vi "motor test 002.vi"() -> ()   [LabVIEW 2019]
uses:
  <vilib>/Platform/TimedLoop/XDataNode/timing_clust.ctl
  <vilib>/Platform/TimedLoop/XDataNode/nitl_modes.ctl
  <vilib>/Platform/TimedLoop/XDataNode/wakeup.ctl
  low level/motor/motor enum.ctl
  <vilib>/platform/TimedLoop/XDataNode/XDataNode.xnode
  low level/motor/motor.lvlib
  <vilib>/Platform/TimedLoop/XDataNode/XDNodeRunTimeDep.lvlib
panel:
  out "E":dbl
  out "Waveform Chart 2":dbl(graph)
  in  "PID gains":T1={"proportional gain (Kc)"=1800.0, "integral time (Ti, min)"=0.0, "derivative time (Td, min)"=0.012}
  out "Waveform Chart":dbl(graph)
  in  "speed RPM":dbl
  in  "reset":bool
  in  "Stop":bool
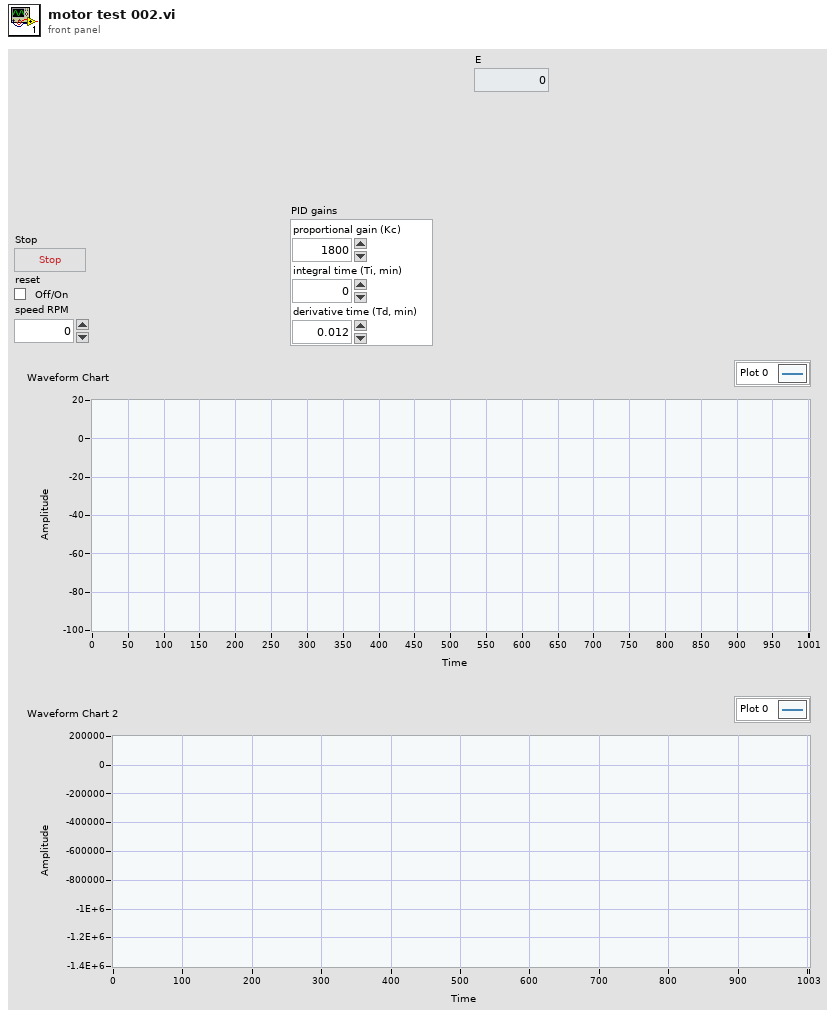
[diagram p1: front panel]
types:
  T1 = cluster{"proportional gain (Kc)":dbl, "integral time (Ti, min)":dbl, "derivative time (Td, min)":dbl}
  T2 = typedef "XDNodeRunTimeDep.lvlib/timing_clust.ctl" = cluster{"Expected End [f-1]":u64, "Actual End [f-1]":u64, "Finished Late? [f-1]":bool, "Expected End [i-1]":u64, "Actual End [i-1]":u64, "Finished Late? [i-1]":bool, "Expected Start [i]":u64, "Actual Start [i]":u64, "Expected Start [f]":u64, "Actual Start [f]":u64, "Source Name":string, "Structure Name":string, "Period":i64, "Deadline":i64, "Offset":i64, "Start":i64, "Priority":i32, "Timeout":i32, "Mode":T3, "Wakeup Reason":T4, "Error":errorcluster, "Source Type":string, "Secondary Source Type":string, "Global End Time":u64, "Global Start Time":u64, "Frame Duration":u64, "Iteration Duration":u64, "Assigned CPU":i32, "I/O Scan Engine Mode":u32}
  T3 = typedef "XDNodeRunTimeDep.lvlib/nitl_modes.ctl" = enum32{"No Change", "Process missed periods, maintain original phase", "Discard missed periods, maintain original phase", "Process missed periods, ignore original phase", "Discard missed periods, ignore original phase"}
  T4 = typedef "XDNodeRunTimeDep.lvlib/wakeup.ctl" = enum32{"Normal", "Aborted", "Asynchronous wakeup", "Timing source error", "Timed loop error", "Timeout"}
  T5 = typedef "my FPGA lib.lvlib/motor.lvlib/motor enum.ctl" = enum16{"M1", "M2", "M3", "M4"}
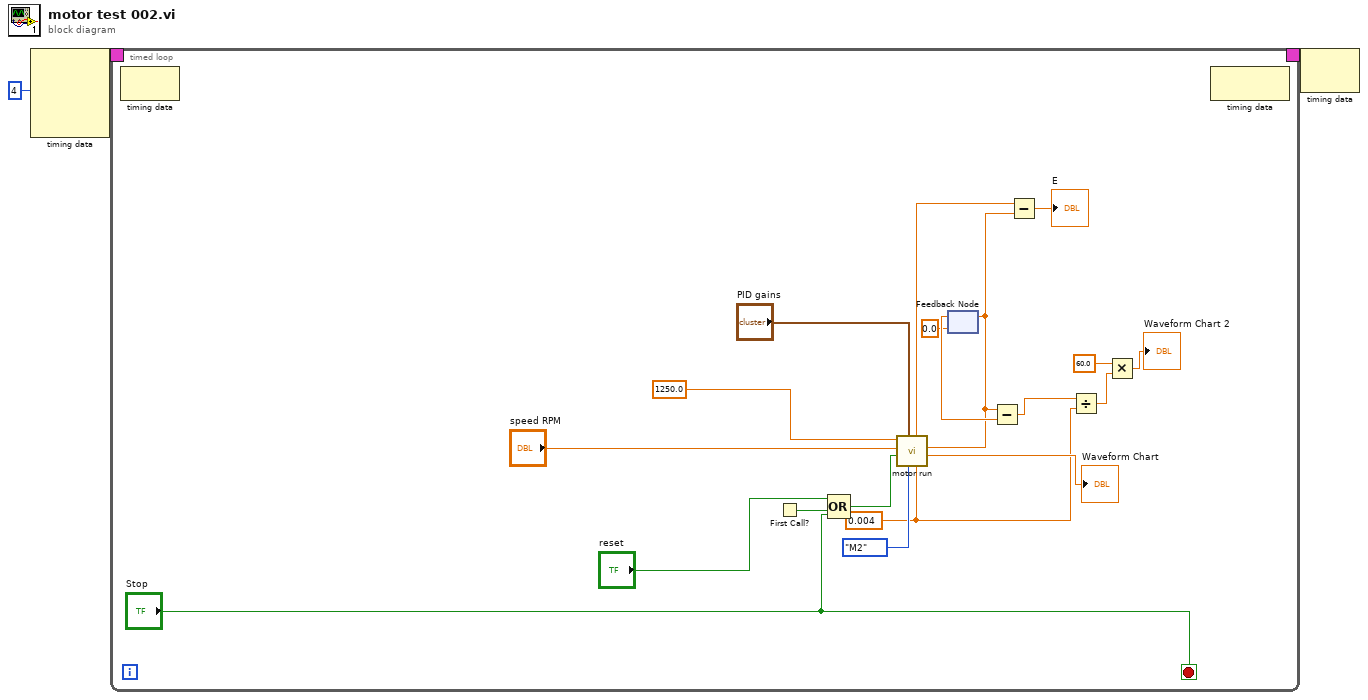
[diagram p0: block diagram]
diagram:
  n1 = node-c288(i64 4 ("Period")) -> (w3:T2)  [unwired: 3 in]
  n2 = timed-loop {
    timing: w3 -> [_]
    timing-out: [_] -> w2
    stop <- "Stop" stop-if-true
    w13 = 0.004 ("dt(s)")
    n3 = node-c288() -> ()  [unwired: 1 in, 1 out]
    n4 = First Call?() -> (First Call?: T/F=w21:bool)
    n5 = Compound Arithmetic op=OR("reset", w21, "Stop") -> (w19:bool)
    n6 = call "motor run.vi"("dt(s)"=w13, "motor select"=motor_enum."M2", "PID gains"="PID gains", "Reset"=w19, "speed RPM"="speed RPM", "PWM frequence"=1250.0) -> ("output"=→"Waveform Chart":dbl, "encoder"=w5:dbl, "setpoint"=w6:dbl)  [unwired: 2 in, 1 out]
    n7 = feedback-in #1(w5) -> ()
    n8 = feedback #1(0.0) -> (w9:dbl)
    n9 = Subtract(x=w5, y=w9) -> (x-y=w7:dbl)
    n10 = Subtract(x=w6, y=w5) -> (x-y=→"E":dbl)
    n11 = Divide(x=w7, y=w13) -> (x/y=w11:dbl)
    n12 = Multiply(x=60.0, y=w11) -> (x*y=→"Waveform Chart 2":dbl)
    n13 = node-c288() -> ()  [unwired: 1 in, 1 out]
  }
  n14 = node-c288(w2) -> ()  [unwired: 1 out]
